vi "Close.vi"(8 "error in":errorcluster, 11 "Acquire Continuous Waveform Configuration in":refnum<class "DS1054 Base CFG.lvclass">) -> (0 "error out":errorcluster, 3 "Acquire Continuous Waveform Configuration out":refnum<class "DS1054 Base CFG.lvclass">)   [LabVIEW 2023, in "RIGOL DS1054Z.lvlib" / "DS1054 Base CFG.lvclass"]
uses:
  DS1054 Base CFG.lvclass
  Scope VISA/Configuration/Scope VISA CFG.lvclass/Scope VISA CFG.ctl
  DS1054 Base CFG.lvclass/DS1054 Base CFG.ctl
  <instrlib>/RIGOL-DS1054Z-LabVIEW/RIGOL DS1054Z Driver.lvlib
  Scope VISA/Configuration/Scope VISA CFG.lvclass
  D:/git/HAL/Scope VISA/Configuration/Scope VISA CFG.lvclass
  D:/git/HAL/Configuration Base/Configuration Base.lvclass
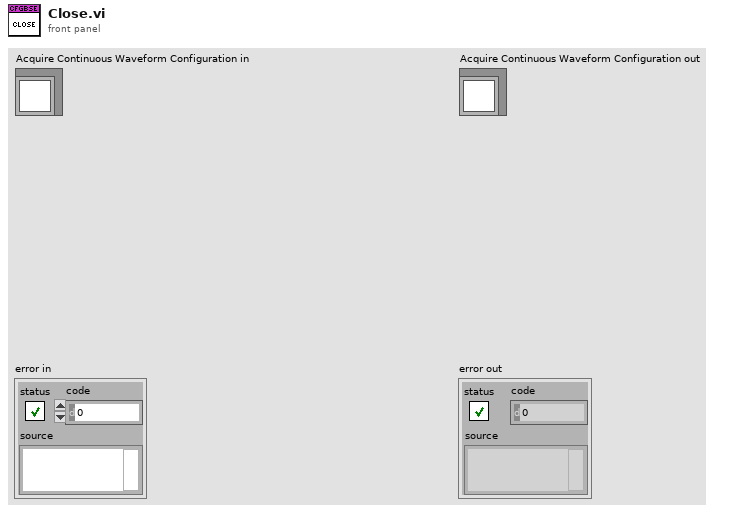
[diagram p1: front panel]
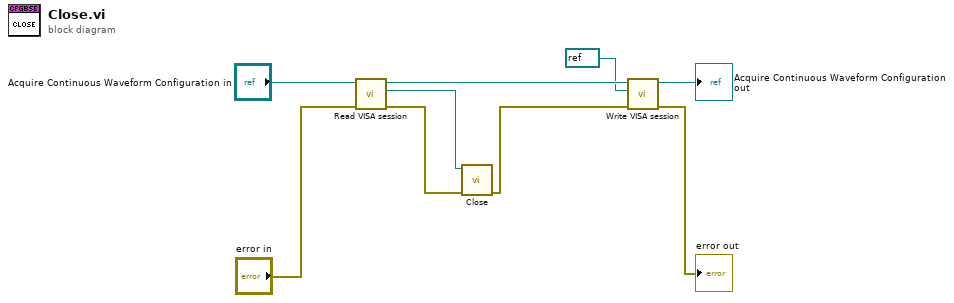
[diagram p0: block diagram]
diagram:
  n1 = call "Read VISA session.vi"("error in (no error)"="error in", "Scope VISA CFG in"="Acquire Continuous Waveform Configuration in") -> ("error out"=w7:errorcluster, "VISA session"=w5:refnum<visa-resource-name>, "Scope VISA CFG out"=w3:refnum<class "DS1054 Base CFG.lvclass">)  [unwired: 7 in]
  n2 = call <instrlib>:"Close.vi"("error in (no error)"=w7, "VISA resource name"=w5) -> ("error out"=w8:errorcluster)  [unwired: 9 out]
  n3 = call "Write VISA session.vi"("error in (no error)"=w8, "VISA session"=refnum<visa-resource-name> refnum, "Scope VISA CFG in"=w3) -> ("error out"=→"error out":errorcluster, "Scope VISA CFG out"=→"Acquire Continuous Waveform Configuration out":refnum<class "DS1054 Base CFG.lvclass">)  [unwired: 7 in]
